vi "send_data_to_cloud.vi"(8 "HTTP client error":errorcluster, 9 "HTTP client handle":T1, 11 "buffer":string) -> (0 "http client error out":errorcluster, 3 "client handle out":T1)   [LabVIEW 2016]
uses:
  <vilib>/httpClient/ClientHandle.ctl
  <vilib>/httpClient/POSTBuffer.vi
  <vilib>/httpClient/LabVIEWHTTPClient.lvlib
panel:
  out "headers":string
  out "body":string
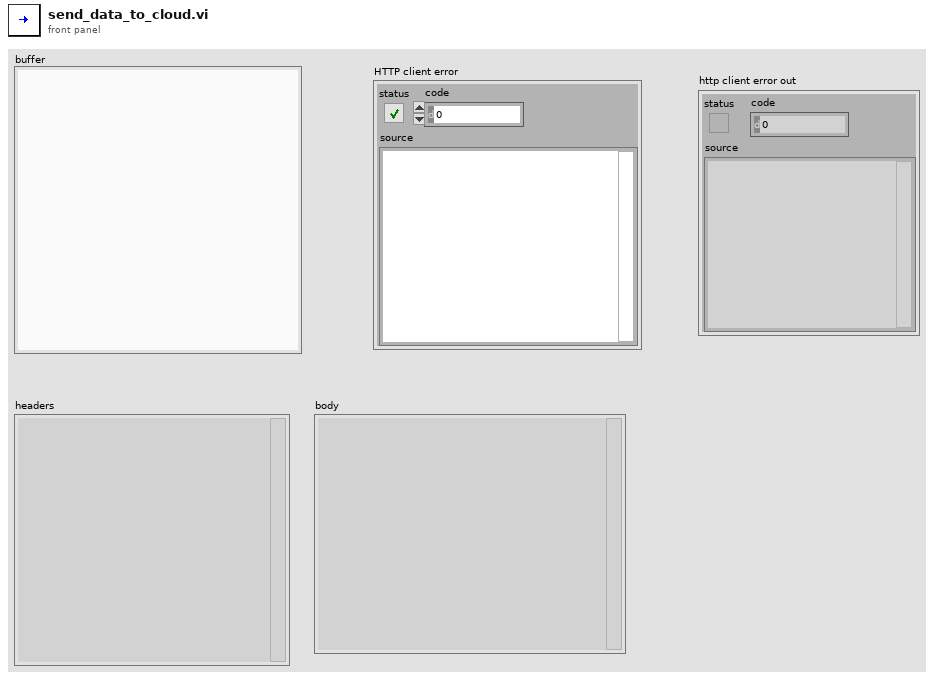
[diagram p1: front panel]
types:
  T1 = typedef "LabVIEWHTTPClient.lvlib/ClientHandle.ctl" = refnum<k1>
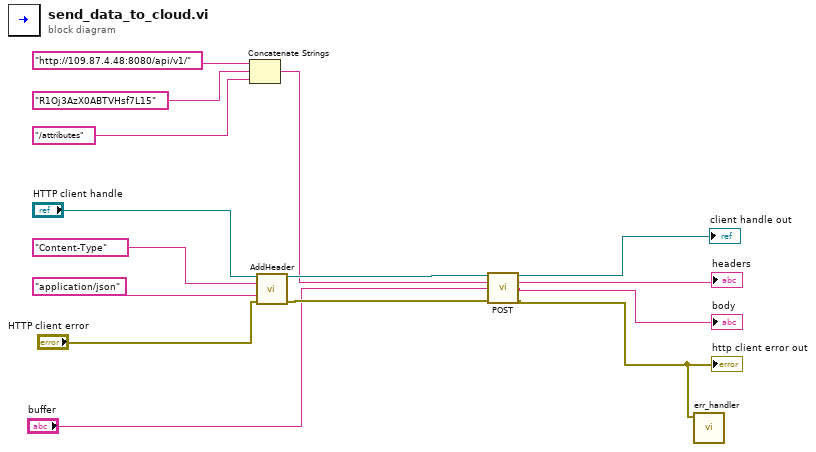
[diagram p0: block diagram]
diagram:
  n1 = Concatenate Strings("http://109.87.4.48:8080/api/v1/" ("url"), "R1Oj3AzX0ABTVHsf7L15" ("string"), "/attributes") -> (w6:string)
  n2 = call <vilib>:"AddHeader.vi"("client handle"="HTTP client handle", "header"="Content-Type", "value"="application/json", "error in (no error)"="HTTP client error") -> ("client handle out"=w11:T1, "error out"=w8:errorcluster)  [unwired: 10 in]
  n3 = call-poly <vilib>:"POST.vi"("client handle"=w11, "url"=w6, "buffer"="buffer", "error in (no error)"=w8) -> ("client handle out"=→"client handle out":T1, "headers"=→"headers":string, "body"=→"body":string, "error out"=w4:errorcluster)  [unwired: 8 in]
  "http client error out" <- w4
  n4 = call "err_handler.vi"("error in (no error)"=w4) -> ()  [unwired: 11 in]
